vi "setOffset.vi"(8 "error in (no error)":errorcluster, 10 "Offset Mode":T1=enum."Remove", 11 "Instrument.LockinAPI in":refnum<class "Instrument.LockinAPI.lvclass">) -> (0 "error out":errorcluster, 3 "Instrument.LockinAPI out":refnum<class "Instrument.LockinAPI.lvclass">)   [LabVIEW 2019, in "Instrument.LockinAPI.lvclass"]
doc: "API to put lockin into IV mode.\n\nIf address=\"\", this API reads from localhost\nIf address is remote lockin, you need to add this computer to allowed whitelist on the lockin computer you are trying to access."
uses:
  Instrument.LockinAPI.lvclass
  Typedefs/Offset Mode--Enum.ctl
  C:/Users/patrick/Documents/GitHub/Instrument-Framework/lvsrc/Instrument/Instrument.lvclass
  Typedefs/API/LockinAPI.Commands--Enum.ctl
  dce59797-926e-44ff-adbc-0402ea62d6fc.vi
  dce59797-926e-44ff-adbc-0402ea62d6fc.vi/6c427a7e-cd5c-4300-8723-7186dccd9928.vi
  dce59797-926e-44ff-adbc-0402ea62d6fc.vi/6c427a7e-cd5c-4300-8723-7186dccd9928.vi/4a0da7cb-6a92-49c7-aca2-2655808a1a6b.vi
  dce59797-926e-44ff-adbc-0402ea62d6fc.vi/6c427a7e-cd5c-4300-8723-7186dccd9928.vi/48c53313-547f-467c-bd73-116b29bc8401.vi
  dce59797-926e-44ff-adbc-0402ea62d6fc.vi/6c427a7e-cd5c-4300-8723-7186dccd9928.vi/41657c35-5942-4e8e-8d0c-37fd14c99172.vi
  <vilib>/JDP Science/JSONtext/Make JSON Array.vi
  dce59797-926e-44ff-adbc-0402ea62d6fc.vi/6c427a7e-cd5c-4300-8723-7186dccd9928.vi/48c53313-547f-467c-bd73-116b29bc8401.vi/aa2431a5-e0c8-442b-a6c1-998aedc5554b.vi
  dce59797-926e-44ff-adbc-0402ea62d6fc.vi/6c427a7e-cd5c-4300-8723-7186dccd9928.vi/41657c35-5942-4e8e-8d0c-37fd14c99172.vi/a3a6f6cc-df23-4589-bc69-c5991e590a83.vi
  dce59797-926e-44ff-adbc-0402ea62d6fc.vi/6c427a7e-cd5c-4300-8723-7186dccd9928.vi/41657c35-5942-4e8e-8d0c-37fd14c99172.vi/5c9bfcd1-3db9-4882-b6dc-3d62541ee820.vi
  Instrument/API/Enum to String.vi
  Instrument/Private/Get RC Connection Status.vi
  <vilib>/JDP Science/JSONtext/Variant to JSON Text.vi
  <vilib>/JDP Science/JSONtext/support/Format JSON Array Text.vi
  Instrument/API/Send and Receive.vi
  <vilib>/JDP Science/JSONtext/JSON text to Variant.vi
  <vilib>/Utility/Data Type/Get Type Information.vi
  <vilib>/JDP Science/JSONtext/LVClass Serializer/JSONtext LVClass Serializer.lvclass
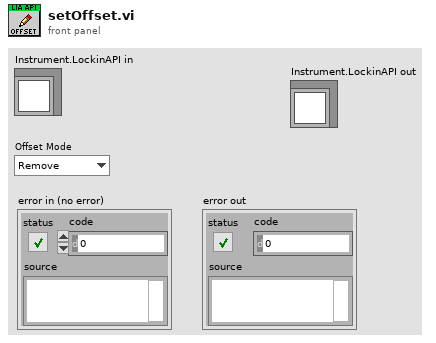
[diagram p1: front panel]
types:
  T1 = typedef "Instrument.LockinAPI.lvclass/Offset Mode--Enum.ctl" = enum16{"Measure", "Remove"}
  T2 = typedef "Instrument.LockinAPI.lvclass/LockinAPI.Commands--Enum.ctl" = enum16{"setAI", "setAO", "setAO_Amplitude", "setAO_DC", "setAO_Frequency", "setAO_Phase", "setAO_Function", "setAO_I+", "setREF", "setREF_Frequency", "setREF_Phase", "setREF_TC", "setREF_Roll-Off", "setDAQ", "setSampling", "setOffset", "setState", "getState", "getAO", "getAI", "getResults", "getSampling", "getAOconfig", "getREFconfig", "setInputGain", "setOutputGain", "getInputGain", "getOutputGain", "setSamplingMode", "getSamplingMode", "setSweep", "setSweepTime", "setSweepTable", "getStatus", "getSweepResults", "getSweepWaveforms", "startSweep", "stopSweep", "setAUX", "getAUX"}
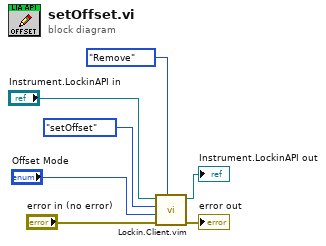
[diagram p0: block diagram]
diagram:
  n1 = call "Lockin.Client.vim"("Data Out type"=Offset_Mode--Enum."Remove" ("Offset Mode"), "error in (no error)"="error in (no error)", "Data"="Offset Mode", "Command"=LockinAPI.Commands--Enum."setOffset", "Instrument.LockinAPI in"="Instrument.LockinAPI in") -> ("error out"=→"error out":errorcluster, "Instrument.LockinAPI out"=→"Instrument.LockinAPI out":refnum<class "Instrument.LockinAPI.lvclass">)  [unwired: 4 in, 1 out]
